vi "Untitled 5.vi"() -> ()   [LabVIEW 2019]
uses:
  <vilib>/eio/EIONode/EIONode.xnode
  <vilib>/rvi/eio/common/nirviEmuTemplateMethod_errors.vi
panel:
  out "Count1":u32
  out "Count0":u32
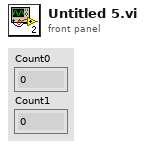
[diagram p1: front panel]
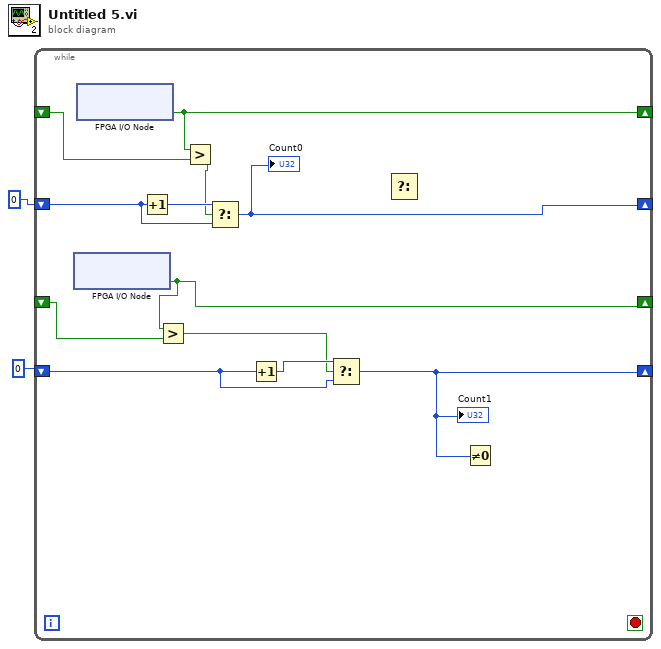
[diagram p0: block diagram]
diagram:
  n1 = while {
    shift-right: [w14] -> _
    shift-left: _ -> [w13]
    shift-right: [w3] -> _
    shift-left: u32 0 ("x") -> [w11]
    shift-right: [w8] -> _
    shift-left: _ -> [w9]
    shift-right: [w4] -> _
    shift-left: u32 0 ("x") -> [w6]
    stop <- _ stop-if-true
    n2 = xnode "FPGA I/O Node"() -> ("Mod8/DI1"=w8:bool)  [unwired: 1 in, 1 out]
    n3 = xnode "FPGA I/O Node"() -> ("Mod8/DI0"=w14:bool)  [unwired: 1 in, 1 out]
    n4 = Increment(x=w11) -> (x+1=w12:u32)
    n5 = Greater?(x=w8, y=w9) -> (0:w5:bool)
    n6 = Greater?(x=w14, y=w13) -> (0:w10:bool)
    n7 = Select(t=w12, s=w10, f=w11) -> (s? t:f=w3:u32)
    "Count0" <- w3
    n8 = Increment(x=w6) -> (x+1=w7:u32)
    n9 = Select(t=w7, s=w5, f=w6) -> (s? t:f=w4:u32)
    "Count1" <- w4
    n10 = Select() -> ()  [unwired: 3 in, 1 out]
    n11 = Not Equal To 0?(x=w4) -> ()  [unwired: 1 out]
  }
